vi "Wiimote Write Data.vi"(7 "Address Space":T1 items=["EEPROM Memory"=0, "Control Register"=4], 8 "error in":errorcluster, 9 "pReportBuffer in":u8[](array[numeric]) format="%02x", 10 "Offset":u32 format="%06x", 11 "hWiimoteHandle in":u32 format="%08x") -> (0 "error out":errorcluster, 3 "hWiimoteHandle out":u32 format="%08x")   [LabVIEW 2010]
uses:
  Wiimote Address Space.ctl
  Wiimote Reporting Mode.ctl
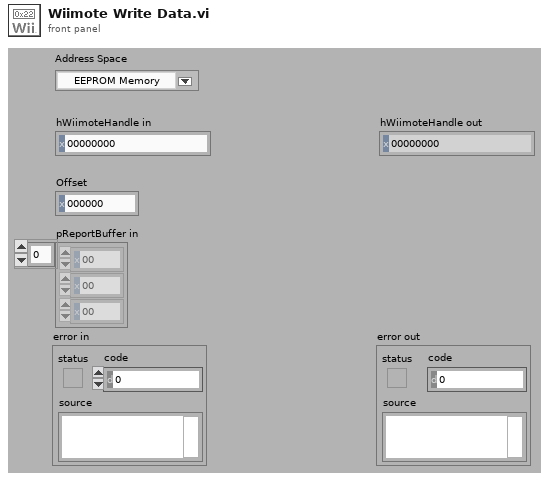
[diagram p1: front panel]
types:
  T1 = typedef "Wiimote Address Space.ctl" = u8
  T2 = typedef "Wiimote Reporting Mode.ctl" = u8
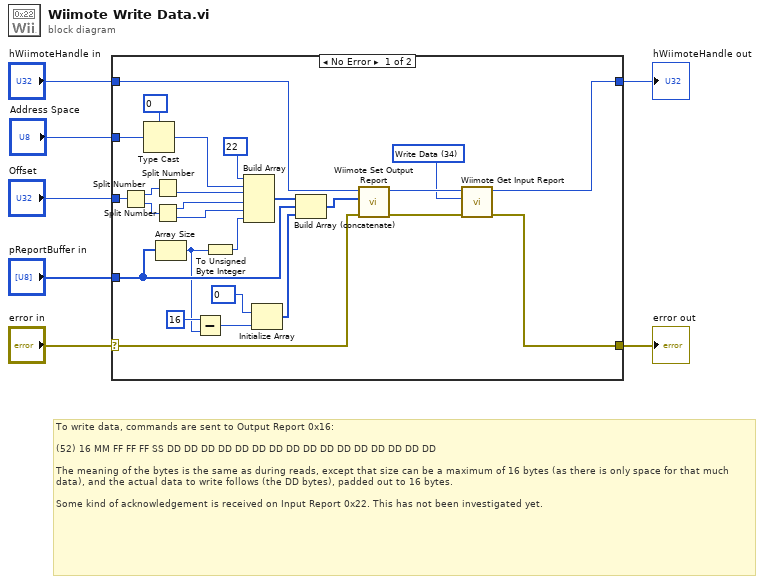
[diagram p0: block diagram]
diagram:
  # "To write data, commands are sent to Output Report 0x16:\n\n(52) 16 MM FF FF FF SS DD DD DD DD DD DD DD DD DD DD DD DD DD DD DD DD\n\nThe meaning of the bytes is the same as during reads, except that size can be a maximum of 16 bytes (as there is only space for that much data), and the actual data to write follows (the DD bytes), padded out to 16 bytes.\n\nSome kind of acknowledgement is received on Input Report 0x22. This has not been investigated yet."
  n1 = case shown="No Error" "error in" {
    selector: "error in" -> [w17 w34]
    tunnel: [w33 w34] -> w7
    tunnel: "hWiimoteHandle in" -> [w32 w35]
    tunnel: [w31 w35] -> w5
    tunnel: "Offset" -> [w25 _]
    tunnel: "pReportBuffer in" -> [w24 _]
    tunnel: "Address Space" -> [w15 _]
    frame No Error {
      w20 = T2 34 items=["Status Information"=32, "Read Data"=33, "Write Data"=34, "Core Buttons"=48, "Core Buttons and Accelerometer"=49, "Core Buttons with 8 Extension bytes"=50, "Core Buttons and Accelerometer with 12 IR bytes"=51, "Core Buttons with 19 Extension bytes"=52, "Core Buttons and Accelerometer with 16 Extension Bytes"=53, "Core Buttons with 10 IR bytes and 9 Extension Bytes"=54, "Core Buttons and Accelerometer with 10 IR bytes and 6 Extension Bytes"=55] ("bInputReport")
      n2 = Split Number(x=w25) -> (hi(x)=w30:u16, lo(x)=w29:u16)
      n3 = Type Cast(type=u8 0, x=w15) -> (*(type *) &x=w14:u8)
      n4 = Split Number(x=w30) -> (lo(x)=w27:u8)  [unwired: 1 out]
      n5 = Split Number(x=w29) -> (hi(x)=w26:u8, lo(x)=w28:u8)
      n6 = Array Size(array=w24) -> (size(s)=w12:i32)
      n7 = Subtract(x=16 ("y"), y=w12) -> (x-y=w11:i32)
      n8 = To Unsigned Byte Integer(number=w12) -> (unsigned 8bit integer=w18:u8)
      n9 = Build Array(u8 22, w14, w27, w26, w28, w18) -> (w19:u8[])
      n10 = Initialize Array(u8 0, w11) -> (w10:u8[])
      n11 = Build Array (concatenate)(w19, w24, w10) -> (w9:u8[])
      n12 = call "Wiimote Set Output Report.vi"("error in"=w17, "pReportBuffer in"=w9, "hWiimoteHandle in"=w32) -> ("error out"=w22:errorcluster, "hWiimoteHandle out"=w23:u32)  [unwired: 7 in]
      n13 = call "Wiimote Get Input Report.vi"("error in"=w22, "bInputReport"=w20, "hWiimoteHandle in"=w23) -> ("error out"=w33:errorcluster, "hWiimoteHandle out"=w31:u32)  [unwired: 6 in, 1 out]
    }
    frame Error {
    }
  }
  "error out" <- w7
  "hWiimoteHandle out" <- w5
